vi "autoDataPaths.vi"() -> ()   [LabVIEW 2017]
uses:
  <vilib>/regexp/Match Regular Expression.xnode
panel:
  out "concatenated string":string
  out "dup path":path
  out "file or folder exists?":bool
  out "filenames":string[](array[string])
  out "output-data-path":path
  out "output-data-name":string
  in  "overwrite":bool
  out "date string":string
  out "metaIn-path":path
  out "dataOutfolder":path
  out "dataIn-path":path
  in  "select pattern":u16(ring) items=["raster_scan_512pix_5mic_01Hz.csv", "raster_scan_512pix_5mic_1.00e-01Hz.csv"]
  in  "stop":bool
  in  "select size":u16(ring) items=["20microns", "5microns"]
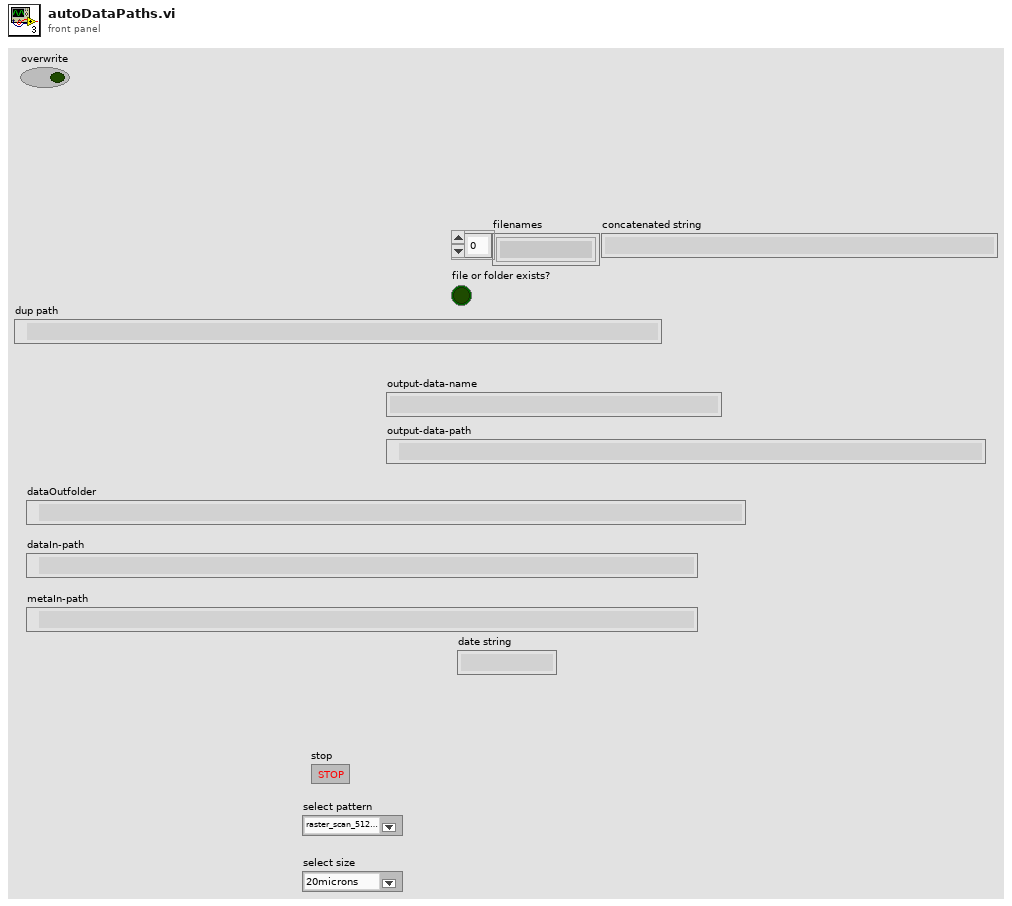
[diagram p1: front panel]
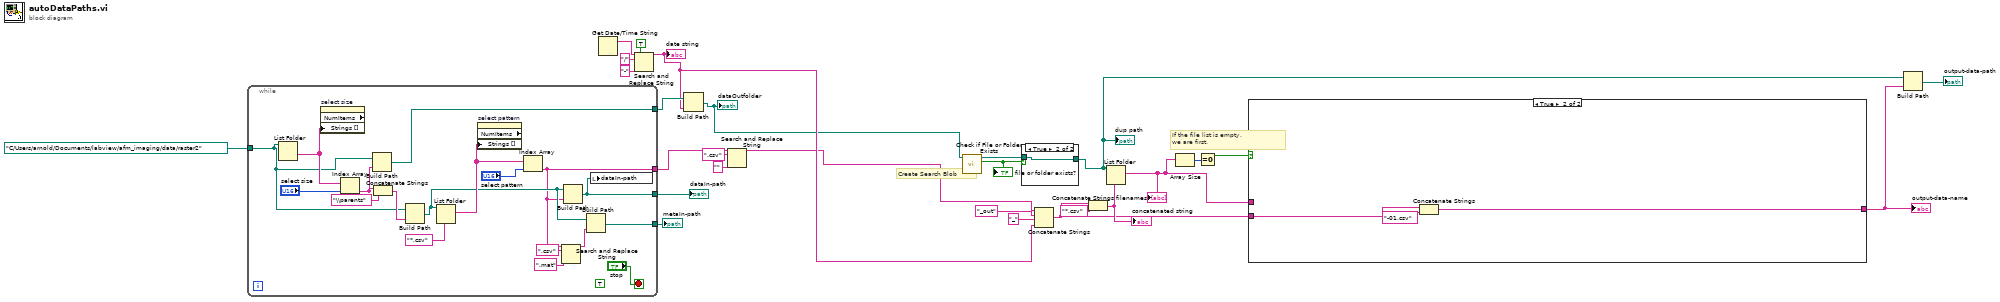
[diagram p0: block diagram]
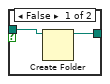
[diagram p2: hidden frame]
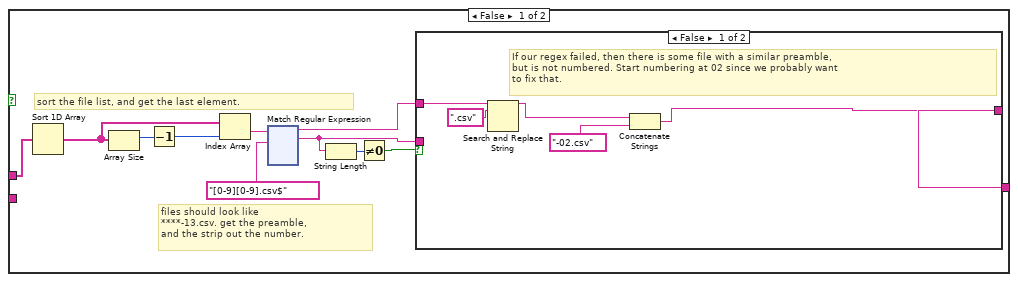
[diagram p3: hidden frame]
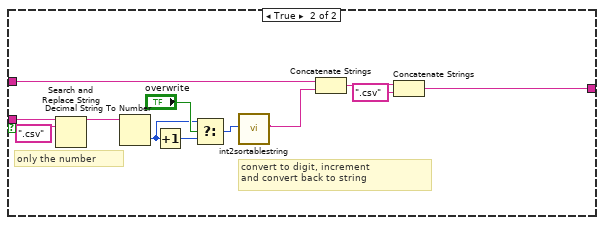
[diagram p4: hidden frame]
diagram:
  # "If the file list is empty,\nwe are first."
  # "Create Search Blob"
  n1 = while {
    tunnel: path "C:/Users/arnold/Documents/labview/afm_imaging/data/raster2" -> [w36]
    tunnel: [w39] -> w26
    tunnel: [w35] -> w20
    tunnel: [w30] -> w25
    tunnel: [w29] -> w10
    stop <- "stop" stop-if-true
    (unwired) TRUE
    n2 = List Folder(path=w36) -> (folder names=w44:string[])  [unwired: 3 in, 3 out]
    n3 = property on="select size" class="Ring (strict)" props=["NumItems", "Strings []"]("Strings []"=w44) -> ()  [unwired: 2 in, 3 out]
    n4 = Index Array(array=w44, index="select size") -> (element=w37:string)
    n5 = Build Path(base path=w36, name or relative path=w37) -> (appended path=w35:path)
    n6 = Concatenate Strings(w37, "\\parents" ("string")) -> (w42:string)
    n7 = Build Path(base path=w36, name or relative path=w42) -> (appended path=w34:path)
    n8 = List Folder(path=w34, pattern="*.csv") -> (filenames=w41:string[])  [unwired: 2 in, 3 out]
    n9 = property on="select pattern" class="Ring (strict)" props=["NumItems", "Strings []"]("Strings []"=w41) -> ()  [unwired: 2 in, 3 out]
    n10 = Index Array(array=w41, index="select pattern") -> (element=w29:string)
    n11 = Search and Replace String(input string=w29, search string=".csv", replace string=".mat" ("replace string (\"\")")) -> (result string=w31:string)  [unwired: 5 in, 3 out]
    n12 = Build Path(base path=w34, name or relative path=w29) -> (appended path=w39:path)
    n13 = Build Path(base path=w34, name or relative path=w31) -> (appended path=w30:path)
    n14 = local write "dataIn-path"(w39) -> ()
  }
  "dataIn-path" <- w26
  "metaIn-path" <- w25
  n15 = Get Date/Time String() -> (date string=w24:string)  [unwired: 3 in, 1 out]
  n16 = Search and Replace String(replace all?=TRUE ("replace all? (F)"), input string=w24, search string="/", replace string="-" ("replace string (\"\")")) -> (result string=w7:string)  [unwired: 4 in, 3 out]
  "date string" <- w7
  n17 = Build Path(base path=w20, name or relative path=w7) -> (appended path=w6:path)
  "dataOutfolder" <- w6
  n18 = Search and Replace String(input string=w10, search string=".csv", replace string="" ("replace string (\"\")")) -> (result string=w1:string)  [unwired: 5 in, 3 out]
  n19 = call <vilib>:"Check if File or Folder Exists.vi"("path"=w6) -> ("file or folder exists?"=w5:bool, "dup path"=w4:path)  [unwired: 8 in, 1 out]
  "file or folder exists?" <- w5
  n20 = case shown="True" w5 {
    tunnel: w4 -> [w47 w48]
    tunnel: [w46 w48] -> w3
    frame False {
      n21 = Create Folder(path (use dialog)=w47) -> (created path=w46:path)  [unwired: 2 in, 2 out]
    }
    frame True {
    }
  }
  "dup path" <- w3
  n22 = Concatenate Strings(w1, "_out" ("replace string (\"\")"), "_", w7) -> (w14:string)
  n23 = Concatenate Strings(w14, "*.csv") -> (w15:string)
  "concatenated string" <- w15
  n24 = List Folder(path=w3, pattern=w15) -> (filenames=w13:string[])  [unwired: 2 in, 3 out]
  "filenames" <- w13
  n25 = Array Size(array=w13) -> (size(s)=w18:i32)
  n26 = Equal To 0?(x=w18) -> (x = 0?=w17:bool)
  n27 = case shown="True" w17 {
    tunnel: w14 -> [_ w191]
    tunnel: [w53 w192] -> w11
    tunnel: w13 -> [w59 _]
    frame False {
      # "files should look like\n****-13.csv. get the preamble,\nand the strip out the number."
      # "sort the file list, and get the last element."
      n28 = Sort 1D Array(array=w59) -> (sorted array=w54:string[])
      n29 = Array Size(array=w54) -> (size(s)=w56:i32)
      n30 = Decrement(x=w56) -> (x-1=w55:i32)
      n31 = Index Array(array=w54, index=w55) -> (element=w58:string)
      n32 = xnode "Match Regular Expression"("input string"=w58, "regular expression"="[0-9][0-9].csv$") -> ("before match"=w52:string, "whole match"=w51:string)  [unwired: 4 in, 3 out]
      n33 = String Length(string=w51) -> (length=w50:i32)
      n34 = Not Equal To 0?(x=w50) -> (x != 0?=w49:bool)
      n35 = case shown="False" w49 {
        tunnel: w51 -> [_ w76]
        tunnel: [w64 w71] -> w53
        tunnel: w52 -> [w61 w70]
        frame False {
          # "If our regex failed, then there is some file with a similar preamble,\nbut is not numbered. Start numbering at 02 since we probably want\nto fix that."
          n36 = Search and Replace String(input string=w61, search string=".csv") -> (result string=w60:string)  [unwired: 6 in, 3 out]
          n37 = Concatenate Strings(w60, "-02.csv" ("string")) -> (w64:string)
        }
        frame True {
          # "convert to digit, increment\nand convert back to string"
          # "only the number"
          n38 = Search and Replace String(input string=w76, search string=".csv") -> (result string=w74:string)  [unwired: 6 in, 3 out]
          n39 = Decimal String To Number(string=w74) -> (number=w65:i32)  [unwired: 2 in, 1 out]
          n40 = Increment(x=w65) -> (x+1=w68:i32)
          n41 = Select(t=w65, s="overwrite", f=w68) -> (s? t:f=w67:i32)
          n42 = call "int2sortablestring.vi"("int"=w67) -> ("tens-sortable-string"=w69:string)  [unwired: 10 in]
          n43 = Concatenate Strings(w70, w69) -> (w73:string)
          n44 = Concatenate Strings(w73, ".csv" ("string")) -> (w71:string)
        }
      }
    }
    frame True {
      n45 = Concatenate Strings(w191, "-01.csv") -> (w192:string)
    }
  }
  "output-data-name" <- w11
  n46 = Build Path(base path=w3, name or relative path=w11) -> (appended path=→"output-data-path":path)
